vi "Path To UTF-8 String.vi"(8 "error in":errorcluster, 11 "Path":path) -> (0 "error out":errorcluster, 3 "UTF-8 String":string)   [LabVIEW 2020, in "G-Image.lvlib"]
doc: "Convert the path input to UTF-8 based on the OS code page. If the input is a string, it is left unchanged."
uses:
  G-Image.lvlib
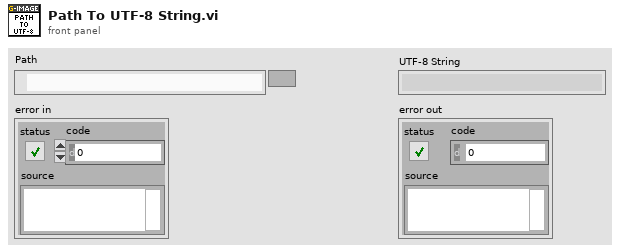
[diagram p1: front panel]
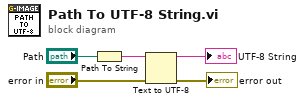
[diagram p0: block diagram]
diagram:
  n1 = Path To String(path="Path") -> (string=w3:string)
  n2 = Text to UTF-8(8:"error in", 11:w3) -> (0:→"error out":errorcluster, 3:→"UTF-8 String":string)  [unwired: 1 in]
